vi "Calculate K and P Kalman.vi"(6 "R Matrix":T1=[[1e-10, 0.0], [0.0, 1e-11]], 7 "Q'=GQG' (Q scalar =1)":T1=[[2.5000000000000003e-17, 5e-13], [5e-13, 1e-08]], 9 "F  Matrix":T1=[[1.0, 0.0001], [0.0, 1.0]], 10 "H Matrix":T1=[[0.0, 1.0], [9.81, 0.0]], 11 "Number of iterations":i32=50) -> (1 "Trace of P":dbl[](array[numeric])=[1.0100103864374432e-08, 1.0099071241173679e-08, 1.0099053913968777e-08, 1.0099045278716121e-08, 1.0099040091621489e-08, 1.0099036631131875e-08, 1.0099034158204801e-08, 1.0099032302912134e-08, 1.0099030859577277e-08, 1.0099029704721776e-08, 1.0099028759732476e-08, 1.0099027972181343e-08, 1.0099027305761128e-08, 1.0099026734531537e-08, 1.0099026239465627e-08, 1.0099025806290573e-08, 1.0099025424090118e-08, 1.0099025084372642e-08, 1.0099024780433431e-08, 1.0099024506908094e-08, 1.0099024259453614e-08, 1.0099024034516291e-08, 1.009902382916023e-08, 1.0099023640938665e-08, 1.009902346779618e-08, 1.009902330799346e-08, 1.009902316004879e-08, 1.0099023022692066e-08, 1.0099022894828302e-08, 1.0099022775508486e-08, 1.0099022663906008e-08, 1.0099022559297561e-08, 1.0099022461047493e-08, 1.0099022368594909e-08, 1.0099022281443006e-08, 1.0099022199150157e-08, 1.0099022121322478e-08, 1.0099022047607532e-08, 1.009902197768902e-08, 1.0099021911282272e-08, 1.0099021848130378e-08, 1.0099021788000882e-08, 1.0099021730682973e-08, 1.0099021675984975e-08, 1.0099021623732265e-08, 1.0099021573765388e-08, 1.0099021525938462e-08, 1.0099021480117755e-08, 1.0099021436180465e-08, 1.0099021394013596e-08], 2 "Steady State P matrix":T1=[[2.1207340437053393e-15, 5.148482094242508e-13], [5.148482094242506e-13, 1.0099019273279553e-08]], 3 "Steady State Kalman Predictor Gain matrixx":T1=[[0.0001484820942425092, 0.002054458487530419], [0.9901927327955272, 0.004852302736465919]])   [LabVIEW 2016]
uses:
  <vilib>/Analysis/NI_AALBase.lvlib
  <vilib>/Analysis/baseanly.llb/Real A x B.vi
  <vilib>/Analysis/NI_AALPro.lvlib
  <vilib>/Analysis/7linalg.llb/Real Transpose Matrix.vi
  <vilib>/Analysis/Matrix/NI_Matrix.lvlib
  <vilib>/Analysis/Matrix/Numeric/Add/Add - RM,RM.vi
  <vilib>/Analysis/baseanly.llb/Real Inverse Matrix.vi
  <vilib>/Analysis/_algsub.llb/Real Matrix Trace.vi
  <vilib>/Analysis/Matrix/Numeric/Subtract/Subtract - RM,RM.vi
  <vilib>/Analysis/7linalg.llb/Create Special Real Matrix.vi
  <vilib>/Analysis/Matrix/Numeric/Multiply/Multiply - RM,R.vi
  <vilib>/Analysis/Matrix/Datatypes/RealMatrix.ctl
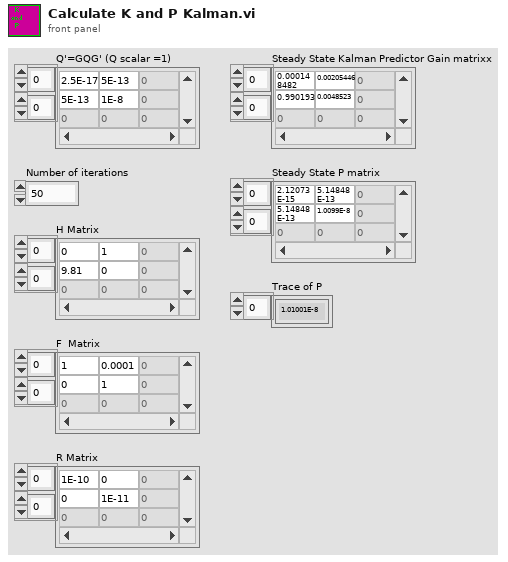
[diagram p1: front panel]
types:
  T1 = typedef "NI_Matrix.lvlib/RealMatrix.ctl" = dbl[][]
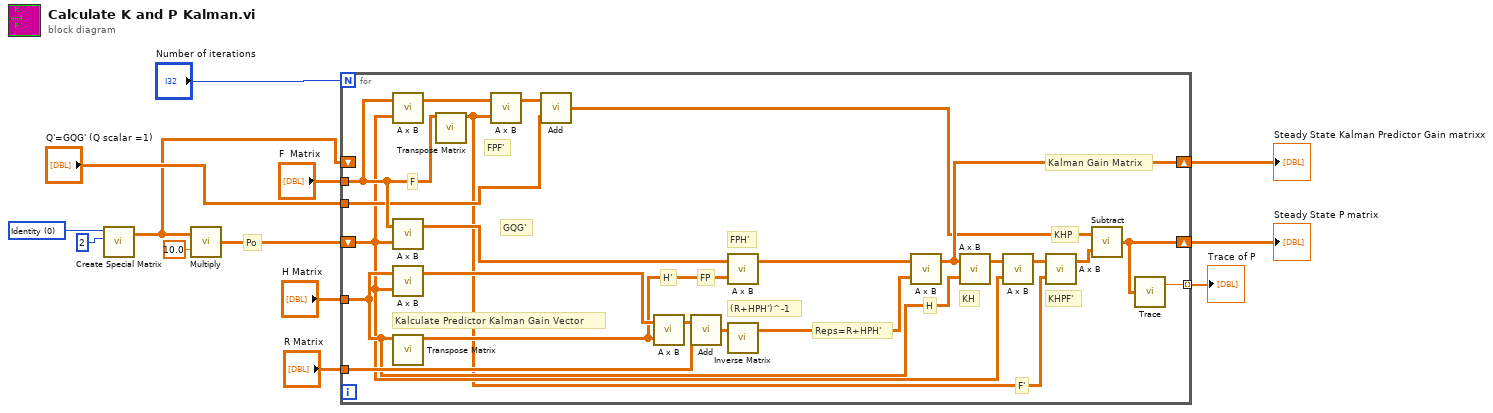
[diagram p0: block diagram]
diagram:
  w2 = 0 items=["Identity", "Diagonal", "Toeplitz", "Vandermonde", "Companion", "Hankel", "Hadamard", "Wilkinson", "Hilbert", "Inverse Hilbert", "Rosser", "Pascal"] ("matrix type")
  # "Po"
  n1 = call-poly <vilib>:"Create Special Matrix.vi"("matrix type"=w2, "matrix size"=2) -> ("Special Matrix"=w11:T1)  [unwired: 3 in, 1 out]
  n2 = call-poly <vilib>:"Multiply.vi"("Real Scalar c"=10.0 ("y"), "Real Matrix A"=w11) -> ("A * c"=w5:T1)
  n3 = for {
    N: "Number of iterations" -> [_]
    shift-right: [w23] -> w9
    shift-left: w5 -> [w17]
    tunnel: "H Matrix" -> [w26]
    tunnel: "R Matrix" -> [w31]
    shift-right: [w27] -> w8
    shift-left: w11 -> [_]
    tunnel: "F  Matrix" -> [w22]
    tunnel: [w24] -> w12 mode=indexing
    tunnel: "Q'=GQG' (Q scalar =1)" -> [w18]
    # "KHPF'"
    # "KHP"
    # "KH"
    # "GQG'"
    # "FPF'"
    # "F'"
    # "F"
    # "Kalman Gain Matrix"
    # "FPH'"
    # "(R+HPH')^-1"
    # "Reps=R+HPH'"
    # "H"
    # "FP"
    # "H'"
    # "Kalculate Predictor Kalman Gain Vector"
    n4 = call-poly <vilib>:"A x B.vi"("B"=w17, "A"=w22) -> ("A x B"=w21:T1)  [unwired: 1 out]
    n5 = call-poly <vilib>:"A x B.vi"("B"=w17, "A"=w22) -> ("A x B"=w35:T1)  [unwired: 1 out]
    n6 = call-poly <vilib>:"A x B.vi"("B"=w17, "A"=w26) -> ("A x B"=w34:T1)  [unwired: 1 out]
    n7 = call-poly <vilib>:"Transpose Matrix.vi"("Input Matrix"=w26) -> ("Matrix Transpose"=w33:T1)  [unwired: 9 in, 1 out]
    n8 = call-poly <vilib>:"Transpose Matrix.vi"("Input Matrix"=w22) -> ("Matrix Transpose"=w15:T1)  [unwired: 9 in, 1 out]
    n9 = call-poly <vilib>:"A x B.vi"("B"=w15, "A"=w21) -> ("A x B"=w20:T1)  [unwired: 1 out]
    n10 = call-poly <vilib>:"Add.vi"("Real Matrix B"=w18, "Real Matrix A"=w20) -> ("A + B"=w19:T1)
    n11 = call-poly <vilib>:"A x B.vi"("B"=w33, "A"=w34) -> ("A x B"=w32:T1)  [unwired: 1 out]
    n12 = call-poly <vilib>:"Add.vi"("Real Matrix B"=w31, "Real Matrix A"=w32) -> ("A + B"=w30:T1)
    n13 = call-poly <vilib>:"A x B.vi"("B"=w33, "A"=w35) -> ("A x B"=w29:T1)  [unwired: 1 out]
    n14 = call-poly <vilib>:"Inverse Matrix.vi"("Input Matrix"=w30) -> ("Inverse Matrix"=w28:T1)  [unwired: 1 in, 1 out]
    n15 = call-poly <vilib>:"A x B.vi"("B"=w28, "A"=w29) -> ("A x B"=w27:T1)  [unwired: 1 out]
    n16 = call-poly <vilib>:"A x B.vi"("B"=w26, "A"=w27) -> ("A x B"=w25:T1)  [unwired: 1 out]
    n17 = call-poly <vilib>:"A x B.vi"("B"=w17, "A"=w25) -> ("A x B"=w16:T1)  [unwired: 1 out]
    n18 = call-poly <vilib>:"A x B.vi"("B"=w15, "A"=w16) -> ("A x B"=w14:T1)  [unwired: 1 out]
    n19 = call-poly <vilib>:"Subtract.vi"("Real Matrix B"=w14, "Real Matrix A"=w19) -> ("A - B"=w23:T1)
    n20 = call-poly <vilib>:"Trace.vi"("Input Matrix"=w23) -> ("trace"=w24:dbl)  [unwired: 1 out]
  }
  "Trace of P" <- w12
  "Steady State P matrix" <- w9
  "Steady State Kalman Predictor Gain matrixx" <- w8
